vi "ConvertForASIO.vi"(10 "bits":i32, 11 "input channel":dbl[](array[numeric])) -> (3 "signal for ASIO":i32[][](array[numeric]))   [LabVIEW 2016]
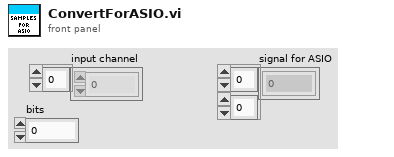
[diagram p1: front panel]
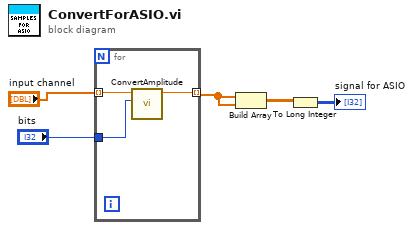
[diagram p0: block diagram]
diagram:
  n1 = for {
    tunnel: "input channel" -> [w8] mode=indexing
    tunnel: [w7] -> w2 mode=indexing
    tunnel: "bits" -> [w6]
    n2 = call "ConvertAmplitude.vi"("bits"=w6, "amplitude [0, 1]"=w8) -> ("generated amplitude [0, 2^(bits - 1) - 1]"=w7:dbl)  [unwired: 9 in]
  }
  n3 = Build Array(w2, w2) -> (w4:dbl[][])
  n4 = To Long Integer(number=w4) -> (32bit integer=→"signal for ASIO":i32[][])
